vi "Set Message Window.vi"(8 "error in (no error)":errorcluster, 11 "wnd":u32) -> (0 "error out":errorcluster, 2 "function return":u32, 3 "wnd out":u32)   [LabVIEW 2014, in "atmcd32d.lvlib"]
doc: "unsigned int WINAPI SetMessageWindow(HWND wnd);"
uses:
  atmcd32d.lvlib
  atmcd32d.dll
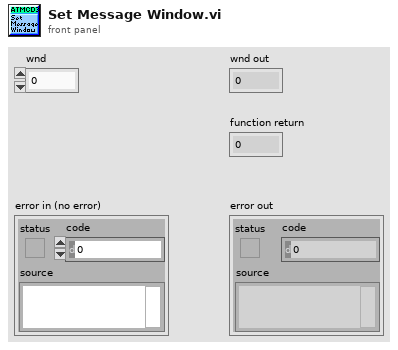
[diagram p1: front panel]
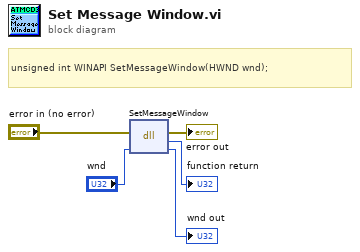
[diagram p0: block diagram]
diagram:
  # "unsigned int WINAPI SetMessageWindow(HWND wnd);"
  n1 = dll-call lib="C:/Users/Bakir/Documents/Lambda2-Testing/lib/Andorlib/atmcd32d.*" fn="SetMessageWindow"(error in="error in (no error)", "wnd"="wnd") -> (error out=→"error out":errorcluster, →"function return":u32, "wnd"=→"wnd out":u32)  [unwired: 2 in, 1 out]
